vi "Bombas.vi"() -> ()   [LabVIEW 2020]
panel:
  out "Bombas":T1
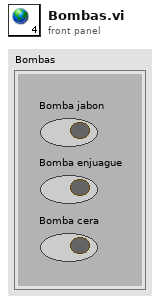
[diagram p1: front panel]
types:
  T1 = cluster{"Bomba jabon":bool, "Bomba enjuague":bool, "Bomba cera":bool}
diagram:
